vi "Resample 1D array.vi"(2 "1D array":dbl[](array[numeric]), 3 "New length":i32=1000) -> (0 "Resampled 1D array":dbl[](array[numeric]))   [LabVIEW 2010]
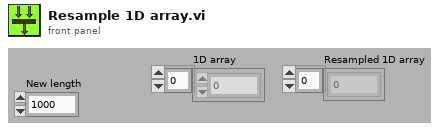
[diagram p1: front panel]
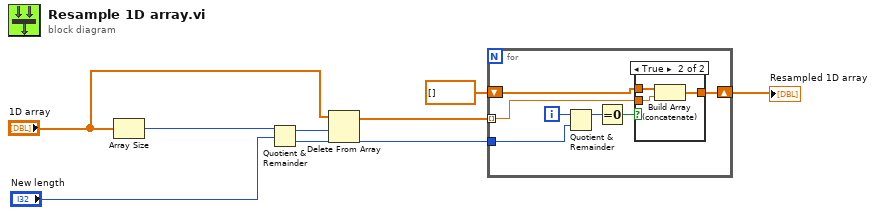
[diagram p0: block diagram]
diagram:
  n1 = Array Size(array="1D array") -> (size(s)=w6:i32)
  n2 = Quotient & Remainder(x=w6, y="New length") -> (x-y*floor(x/y)=w4:i32, floor(x/y)=w1:i32)
  n3 = Delete From Array(array="1D array", length=w4) -> (array with subset deleted=w2:dbl[])  [unwired: 1 in, 1 out]
  n4 = for {
    tunnel: w2 -> [w13] mode=indexing
    shift-right: [w15] -> w7
    shift-left: dbl[] [] ("Y") -> [w14]
    tunnel: w1 -> [w9]
    i -> [w11]
    n5 = Quotient & Remainder(x=w11, y=w9) -> (x-y*floor(x/y)=w12:i32)  [unwired: 1 out]
    n6 = Equal To 0?(x=w12) -> (x = 0?=w10:bool)
    n7 = case shown="True" w10 {
      tunnel: [w16 w19] -> w15
      tunnel: w14 -> [w16 w18]
      tunnel: w13 -> [_ w17]
      frame False {
      }
      frame True {
        n8 = Build Array (concatenate)(w18, w17) -> (w19:dbl[])
      }
    }
  }
  "Resampled 1D array" <- w7
